vi "Transmitter_RSMA - Timer & Modulation Config.vi"() -> ()   [LabVIEW 2022 SP3]
uses:
  <instrlib>/niUSRP/niUSRP Write Tx Data (CDB).vi
panel:
  in  "Iterations":i32=10000
  out "Time(s)":sgl format="%#_4g"
  in  "Alpha":dbl(slide)=0.17500000000000002 step=0.005 scale=0.0..1.0
  in  "Tab Control":enum32{"USRP Parameters", "Transmission"}(tab)
  in  "USRP ControledParameters 2":T1={"Active Antenna"="TX1", "Gain (dB)"=0.0, "Carrier Frequency"=2400000000.0, "IQ Rate"=2000000.0, "Active Channel"="0"} {"IQ Rate" format="%#_6p"; "Carrier Frequency" format="%#_6p"; "Gain (dB)" format="%#_6f"}
  in  "Device selection":refnum<k15>="RIO0"
  in  "stop":bool
  out "Error out":errorcluster
  in  "Modulation parameter":T2
  out "Bits length":i32
  out "Bits length 2":i32
  out "Frame Duration":dbl format="%#_6p"
  out "Coerced Parameters":T3={"IQ Rate"=100000.0, "Carrier  Freq."=100000.0, "Gain"=0.0} {"Gain" format="%#_6f"; "Carrier  Freq." format="%#_6p"; "IQ Rate" format="%#_6p"}
  out "Transmitted Waveform":dbl[](graph)
  in  "Message 2":string="ptua. At vero eos et accusam et justo duo dolores et ea rebum. Stet clita kasd gubergren, no sea takimata sanctus est Lorem ipsum dolor sit amet. Lore"
  in  "Message 1":string="Lorem ipsum dolor sit amet, consetetur sadipscing elitr, sed diam nonumy eirmod tempor invidunt ut labore et dolore magna aliquyam erat, sed diam volu"
  in  "error in (no error)":errorcluster
  # "RSMA Transmitter"
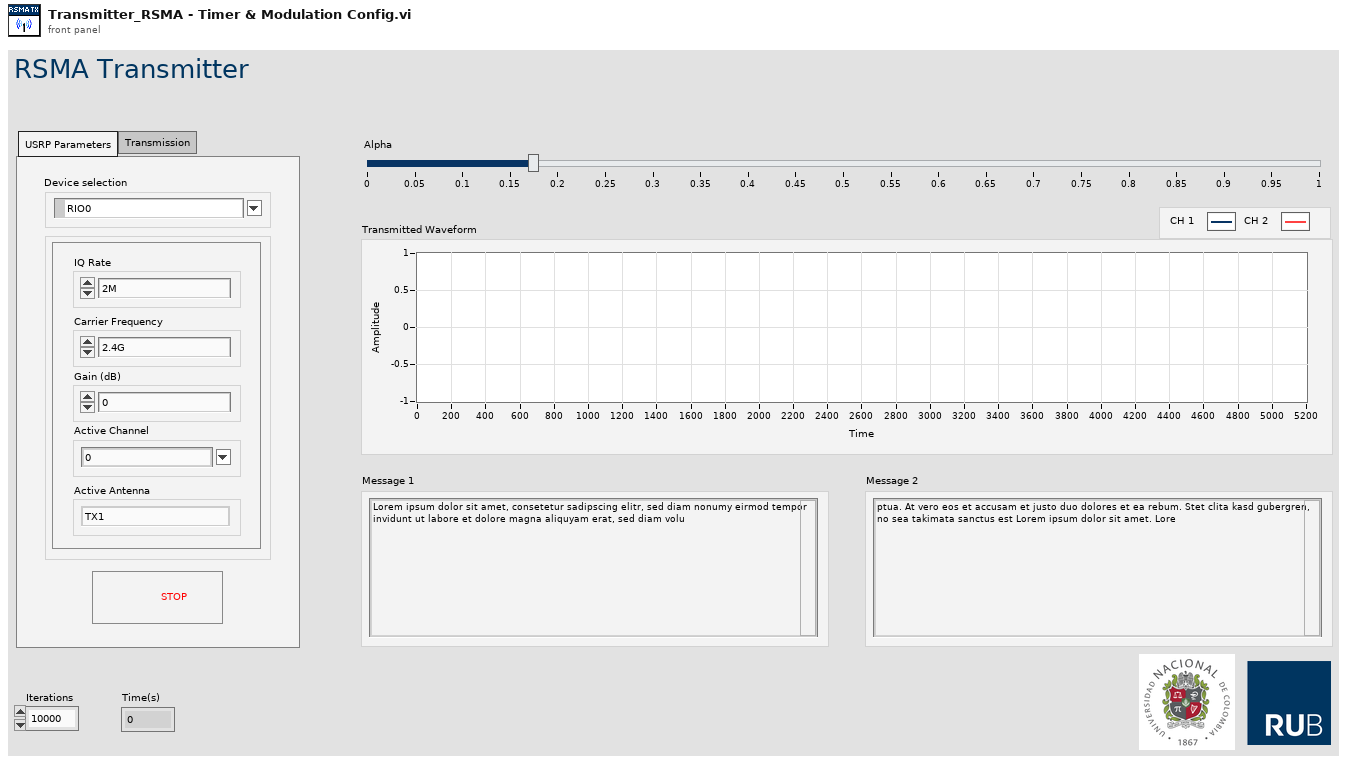
[diagram p1: front panel]
types:
  T1 = cluster{"Active Antenna":string, "Gain (dB)":dbl, "Carrier Frequency":dbl, "IQ Rate":dbl, "Active Channel":string}
  T2 = cluster{"Modulation type":enum16{"QPSK(4QAM)", "64QAM", "16QAM", "BPSK", "BPSK Vertical"}, "BCC rate (k/n)":enum16{"1/2", "2/3", "3/4"}}
  T3 = cluster{"IQ Rate":dbl, "Carrier  Freq.":dbl, "Gain":dbl}
  T4 = cluster{"coerced IQ rate":dbl, "coerced carrier frequency":dbl, "coerced gain":dbl}
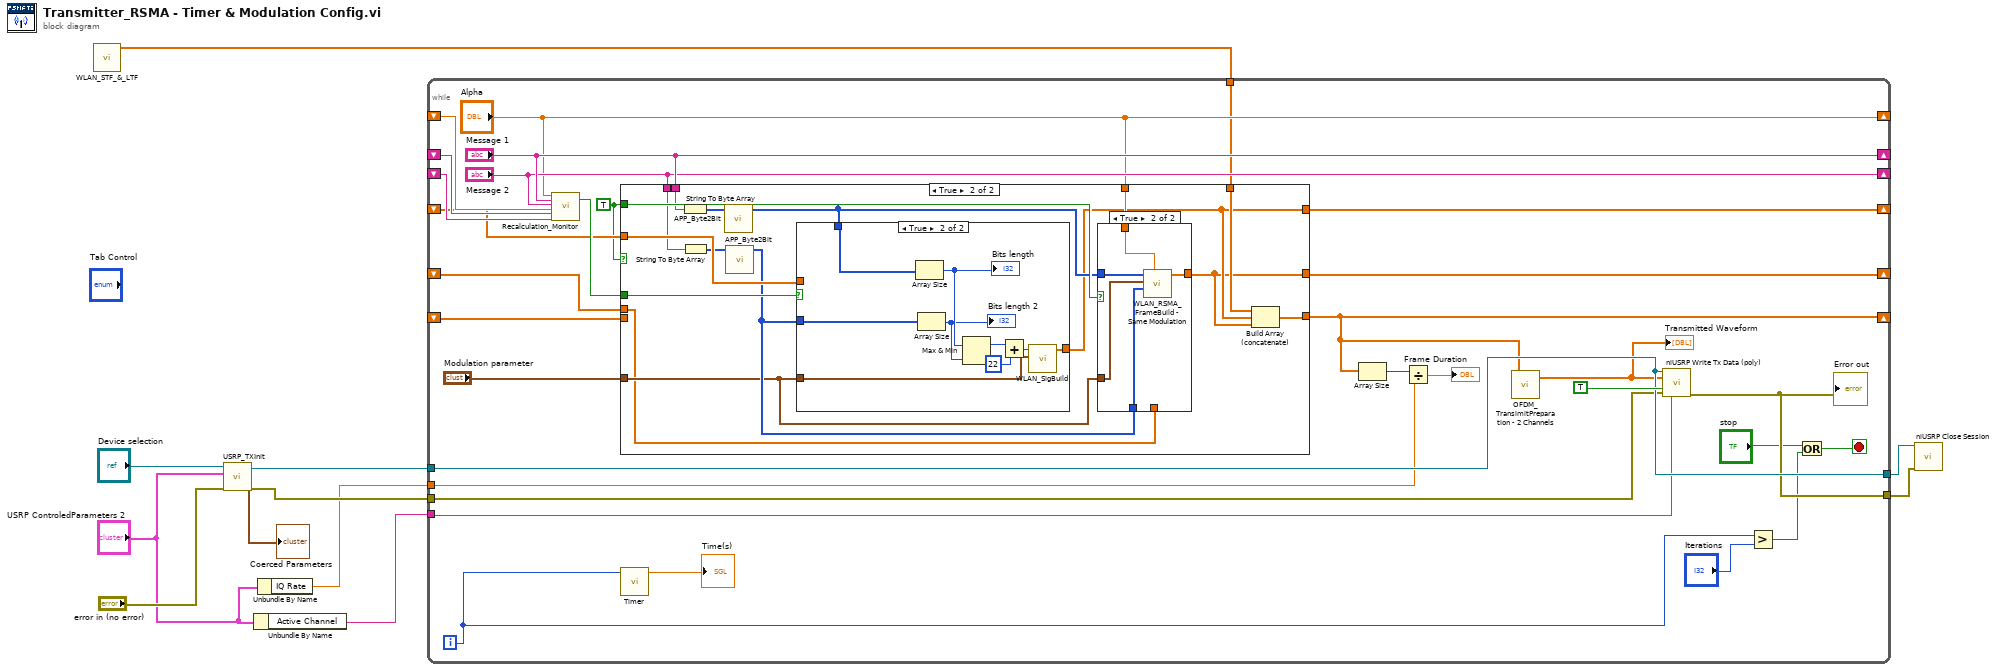
[diagram p0: block diagram]
diagram:
  n1 = call "WLAN_STF_&_LTF.vi"() -> ("STF & LTF"=w1:cdb[])  [unwired: 11 in]
  n2 = call "USRP_TXInit.vi"("device names"="Device selection", "USRP ControledParameters"="USRP ControledParameters 2", "error in (no error)"="error in (no error)") -> ("session handle out"=w10:refnum<k15>, "USRP CoercedParamters"=→"Coerced Parameters":T4, "error out"=w9:errorcluster)  [unwired: 5 in]
  n3 = Unbundle By Name("USRP ControledParameters 2") -> ("Active Channel"=w2:string)
  n4 = Unbundle By Name("USRP ControledParameters 2") -> ("IQ Rate"=w8:dbl)
  n5 = while {
    tunnel: w10 -> [w39]
    tunnel: w9 -> [w22]
    tunnel: w8 -> [w38]
    tunnel: [w39] -> w7
    tunnel: [w37] -> w6
    tunnel: w2 -> [w36]
    shift-right: ["Alpha"] -> _
    shift-left: _ -> [w35]
    shift-right: ["Message 1"] -> _
    shift-left: _ -> [w34]
    shift-right: ["Message 2"] -> _
    shift-left: _ -> [w33]
    shift-right: [w29] -> _
    shift-left: _ -> [w28]
    shift-right: [w26] -> _
    shift-left: _ -> [w25]
    tunnel: w1 -> [w24]
    shift-right: [w21] -> _
    shift-left: _ -> [w23]
    i -> [w17]
    stop <- w14 stop-if-true
    w13 = TRUE
    n6 = call "Recalculation_Monitor.vi"("Alpha"="Alpha", "Message 1"="Message 1", "Message 2"="Message 2", "Alpha old"=w35, "Message 1 old"=w34, "Message 2 old"=w33) -> ("Recalculate SIG"=w32:bool)  [unwired: 11 in, 2 out]
    n7 = case shown="True" w13 {
      tunnel: w32 -> [_ w61]
      tunnel: w13 -> [_ w60]
      tunnel: "Message 1" -> [_ w55]
      tunnel: "Message 2" -> [_ w56]
      tunnel: "Modulation parameter" -> [_ w52]
      tunnel: [w45 w48] -> w29
      tunnel: w28 -> [w45 w59]
      tunnel: "Alpha" -> [_ w51]
      tunnel: [w44 w46] -> w26
      tunnel: w25 -> [w44 w50]
      tunnel: w24 -> [_ w49]
      tunnel: [w43 w47] -> w21
      tunnel: w23 -> [w43 _]
      frame False {
      }
      frame True {
        n8 = String To Byte Array(string=w55) -> (unsigned byte array=w57:u8[])
        n9 = String To Byte Array(string=w56) -> (unsigned byte array=w58:u8[])
        n10 = call "APP_Byte2Bit.vi"("input byte stream"=w57) -> ("output bit stream"=w53:i8[])  [unwired: 10 in]
        n11 = call "APP_Byte2Bit.vi"("input byte stream"=w58) -> ("output bit stream"=w54:i8[])  [unwired: 10 in]
        n12 = case shown="True" w61 {
          tunnel: w52 -> [_ w69]
          tunnel: [w68 w75] -> w48
          tunnel: w59 -> [w68 _]
          tunnel: w54 -> [_ w71]
          tunnel: w53 -> [_ w70]
          frame False {
          }
          frame True {
            n13 = Array Size(array=w70) -> (size(s)=w77:i32)
            "Bits length" <- w77
            n14 = Array Size(array=w71) -> (size(s)=w76:i32)
            "Bits length 2" <- w76
            n15 = Max & Min(x=w77, y=w76) -> (max(x,y)=w73:i32)  [unwired: 1 out]
            n16 = Add(x=w73, y=22) -> (x+y=w74:i32)
            n17 = call "WLAN_SigBuild.vi"("Data bit length"=w74, "Modulation parameter"=w69) -> ("symbols"=w75:cdb[])  [unwired: 7 in, 1 out]
          }
        }
        n18 = case shown="True" w60 {
          tunnel: w54 -> [_ w67]
          tunnel: w53 -> [_ w66]
          tunnel: w52 -> [_ w65]
          tunnel: w51 -> [_ w64]
          tunnel: [w62 w63] -> w46
          tunnel: w50 -> [w62 _]
          frame False {
          }
          frame True {
            n19 = call "WLAN_RSMA_FrameBuild - Same Modulation.vi"("Alpha"=w64, "data in 2"=w67, "Modulation parameter"=w65, "data in"=w66) -> ("output array"=w63:cdb[])  [unwired: 6 in, 1 out]
          }
        }
        n20 = Build Array (concatenate)(w49, w48, w46) -> (w47:cdb[])
      }
    }
    n21 = call "Timer.vi"("index"=w17) -> ("Time(s)"=→"Time(s)":sgl)  [unwired: 10 in]
    n22 = Array Size(array=w21) -> (size(s)=w41:i32)
    n23 = Divide(x=w41, y=w38) -> (x/y=→"Frame Duration":dbl)
    n24 = call "OFDM_TransimitPreparation - 2 Channels.vi"("array"=w21) -> ("output array"=w20:cdb[])  [unwired: 8 in, 2 out]
    "Transmitted Waveform" <- w20
    n25 = call-poly <instrlib>:"niUSRP Write Tx Data (poly).vi"("session handle"=w39, "channel list"=w36, "data"=w20, "end of data?"=TRUE, "error in (no error)"=w22) -> ("error out"=w37:errorcluster)  [unwired: 9 in, 1 out]
    "Error out" <- w37
    n26 = Greater?(x=w17, y="Iterations") -> (0:w15:bool)
    n27 = Or(x="stop", y=w15) -> (x .or. y?=w14:bool)
  }
  n28 = call <instrlib>:"niUSRP Close Session.vi"("session handle"=w7, "error in (no error)"=w6) -> ()  [unwired: 13 in, 1 out]
